vi "GitDiffNowWithHash.vi"(7 "Hash":string, 8 "error in (no error)":errorcluster, 9 "Save Repo Path":path=path "", 10 "Save Cluster":T1 {"Select Layout" items=["Default"]}, 11 "Git exec":string="git") -> (0 "error out":errorcluster, 1 "Save Repo Path Out":path, 2 "Save Cluster Out":T1 {"Select Layout" items=["Default"]}, 3 "Git exec out":string="git", 4 "Diff Output":string, 5 "Differ":bool)   [LabVIEW 2013]
uses:
  TypeDefs/SaveCluster.ctl
  VariableManagerCodes/VariableManager/VariableManager.lvclass
  DeviceVIs/Device/Device.lvclass
  <vilib>/Utility/miscctls.llb/LVStringsAndValuesArrayTypeDef_I32.ctl
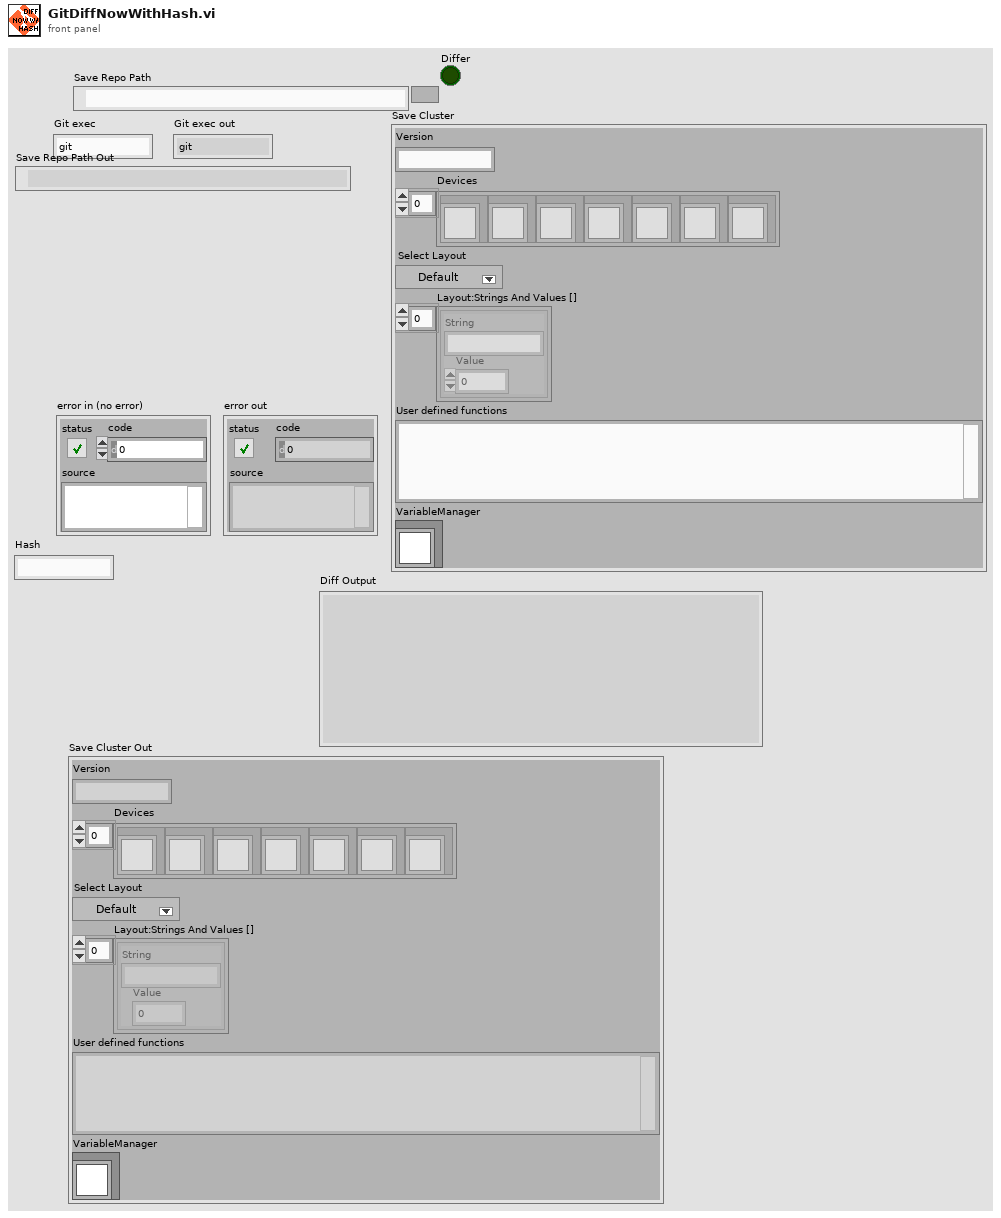
[diagram p1: front panel]
types:
  T1 = typedef "SaveCluster.ctl" = cluster{"Version":string, "Devices":refnum<class "Device.lvclass">[], "Select Layout":i32, "Layout:Strings And Values []":T2, "User defined functions":string, "VariableManager":refnum<class "VariableManager.lvclass">}
  T2 = typedef "LVStringsAndValuesArrayTypeDef_I32.ctl" = cluster{"String":string, "Value":i32}[]
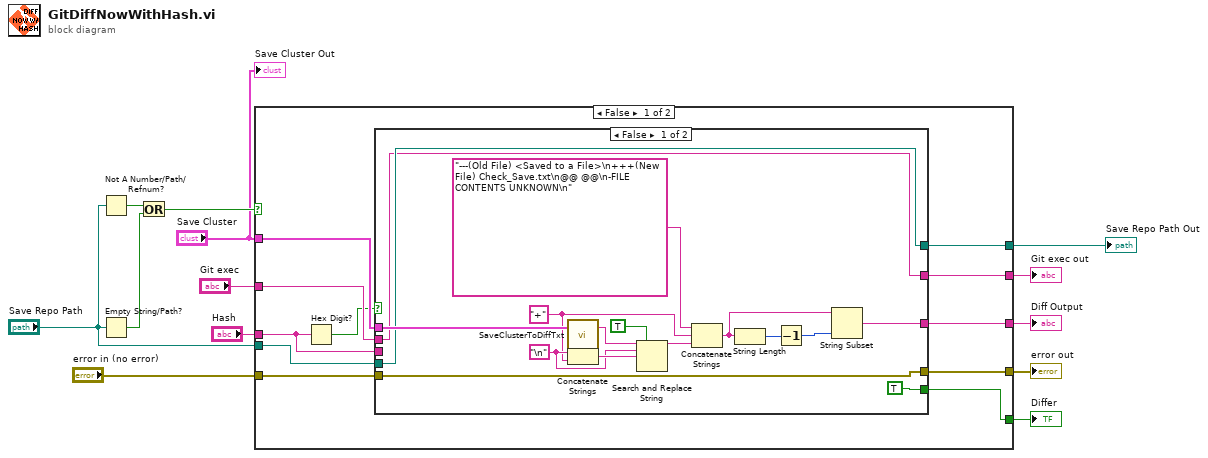
[diagram p0: block diagram]
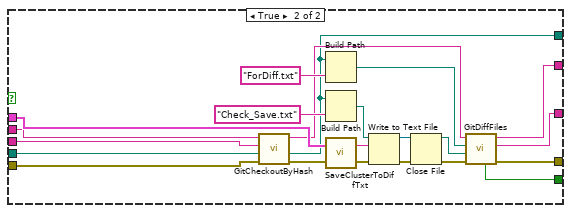
[diagram p2: hidden frame]
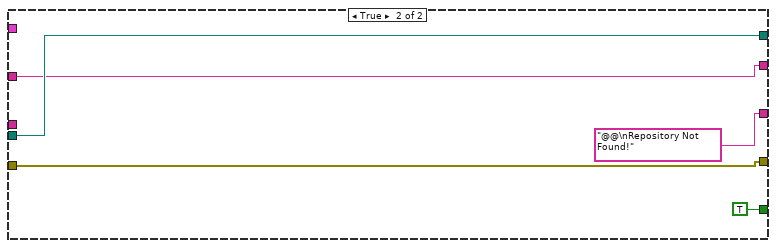
[diagram p3: hidden frame]
diagram:
  n1 = Not A Number/Path/Refnum?(number/path/refnum="Save Repo Path") -> (NaN/Path/Refnum?=w11:bool)
  n2 = Empty String/Path?(string/path="Save Repo Path") -> (empty?=w10:bool)
  n3 = Or(x=w11, y=w10) -> (x .or. y?=w9:bool)
  n4 = case shown="False" w9 {
    tunnel: "error in (no error)" -> [w18 w66]
    tunnel: [w23 w66] -> w6
    tunnel: "Save Repo Path" -> [w19 w65]
    tunnel: [w16 w65] -> w5
    tunnel: "Git exec" -> [w17 w63]
    tunnel: [w24 w63] -> w7
    tunnel: [w22 "@@\nRepository Not Found!" ("Response")] -> w4
    tunnel: [w21 TRUE ("Differ")] -> w3
    tunnel: "Save Cluster" -> [w20 _]
    tunnel: "Hash" -> [w15 _]
    frame False {
      n5 = Hex Digit?(1:w15) -> (0:w14:bool)
      n6 = case shown="False" w14 {
        tunnel: [w35 w55] -> w24
        tunnel: [w37 w54] -> w23
        tunnel: [w25 w53] -> w22
        tunnel: [TRUE ("Differ") w52] -> w21
        tunnel: w20 -> [w40 w50]
        tunnel: w19 -> [w36 w46]
        tunnel: w18 -> [w37 w45]
        tunnel: w17 -> [w35 w44]
        tunnel: [w36 w42] -> w16
        tunnel: w15 -> [_ w41]
        frame False {
          w30 = "\n"
          w29 = "+" ("string")
          n7 = call "SaveClusterToDiffTxt.vi"("Save Cluster"=w40) -> ("DiffText"=w32:string)  [unwired: 2 in]
          n8 = Concatenate Strings(w30, w29) -> (w33:string)
          n9 = Search and Replace String(replace all?=TRUE ("replace all? (F)"), input string=w32, search string=w30, replace string=w33) -> (result string=w31:string)  [unwired: 4 in, 3 out]
          n10 = Concatenate Strings("---(Old File) <Saved to a File>\n+++(New File) Check_Save.txt\n@@ @@\n-FILE CONTENTS UNKNOWN\n" ("string"), w29, w31) -> (w26:string)
          n11 = String Length(string=w26) -> (length=w28:i32)
          n12 = Decrement(x=w28) -> (x-1=w27:i32)
          n13 = String Subset(string=w26, length (rest)=w27) -> (substring=w25:string)  [unwired: 1 in]
        }
        frame True {
          n14 = call "GitCheckoutByHash.vi"("error in (no error)"=w45, "File"=w46, "Hash"=w41, "Git exec"=w44) -> ("error out"=w47:errorcluster, "File out"=w42:path, "Git exec out"=w43:string)  [unwired: 4 in, 1 out]
          n15 = Build Path(base path=w42, name or relative path="ForDiff.txt") -> (appended path=w48:path)
          n16 = Build Path(base path=w42, name or relative path="Check_Save.txt") -> (appended path=w60:path)
          n17 = call "SaveClusterToDiffTxt.vi"("Save Cluster"=w50) -> ("DiffText"=w58:string)  [unwired: 2 in]
          n18 = Write to Text File(file (use dialog)=w60, text=w58, error in=w47) -> (refnum out=w59:refnum<file>, error out=w57:errorcluster)  [unwired: 1 in, 1 out]
          n19 = Close File(refnum=w59, error in=w57) -> (path=w49:path, error out=w56:errorcluster)
          n20 = call "GitDiffFiles.vi"("error in (no error)"=w56, "New File"=w49, "Old File"=w48, "Git exec"=w43) -> ("error out"=w54:errorcluster, "Response"=w53:string, "Git exec out"=w55:string, "Differ"=w52:bool)  [unwired: 3 in, 1 out]
        }
      }
    }
    frame True {
    }
  }
  "Git exec out" <- w7
  "error out" <- w6
  "Diff Output" <- w4
  "Save Repo Path Out" <- w5
  "Differ" <- w3
  "Save Cluster Out" <- "Save Cluster"
